vi "Solver LLB Pre-Check.vi"(8 "error in":errorcluster, 11 "Solver LLB":path) -> (0 "error out":errorcluster, 3 "Issues Detected":string)   [LabVIEW 2020]
uses:
  <vilib>/Utility/traverseref.llb/TRef TravTarget.ctl
  c793339f-25fd-4173-b65a-4e1b08b07bf6.vi
  1ab69464-b1f4-4e58-a4b1-b8e24fb308a9.vi
  <vilib>/Utility/traverseref.llb/VI Scripting - Traverse.lvlib
panel:
  in  "Prohibited Libraries":string[](array[string])=["Skyline", "registry"]
  in  "Prohibited Nodes":string[](array[string])=["Open VI Reference", "Call Library Function Node", "Traverse for GObjects.vi", "TCP Write", "TCP Read", "Call Chain", "Python Node", "Constructor Node", "Automation Open", "System Exec.vi", "Delete", "Librarian Delete.vi", "Delete Directory Recursive.vi", "Read Multiple Elements from Stream", "Read Single Element from Stream", "Write Multiple Elements to Stream", "Write Single Element to Stream", "VISA Write", "VISA Read", "DataSocket Read", "DataSocket Write"]
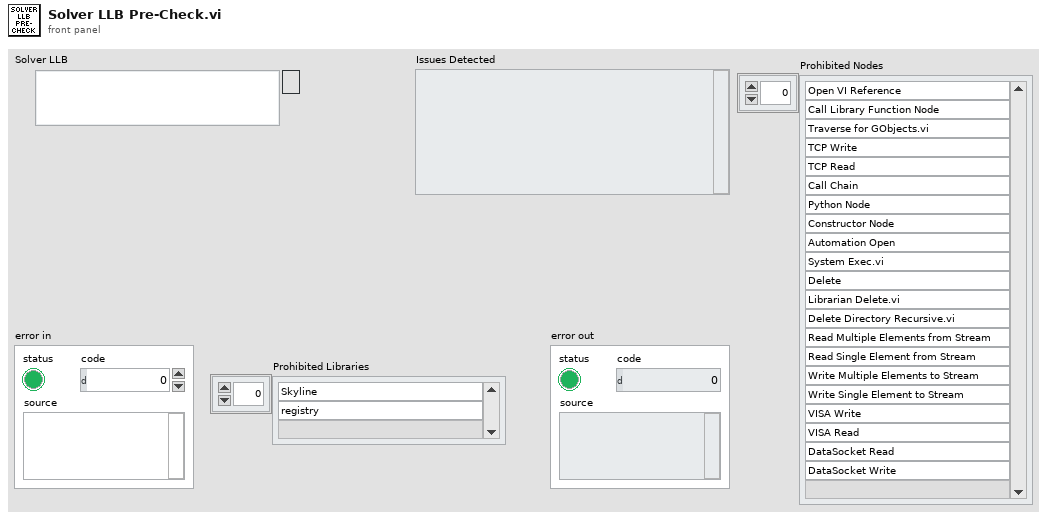
[diagram p1: front panel]
types:
  T1 = enum16{"Initialize", "Password-Protection", "Prohibited Nodes", "Prohibited Libraries", "Close"}
  T2 = enum16{"Initialize", "Password-Protection", "Prohibited Nodes", "Prohibited Libraries", "Close"}[]
  T3 = enum32{"invalid lock state", "Not Locked", "Locked (No Password)", "Password-protected"}
  T4 = typedef "TRef TravTarget.ctl" = enum16{"FP", "BD", "Other"}
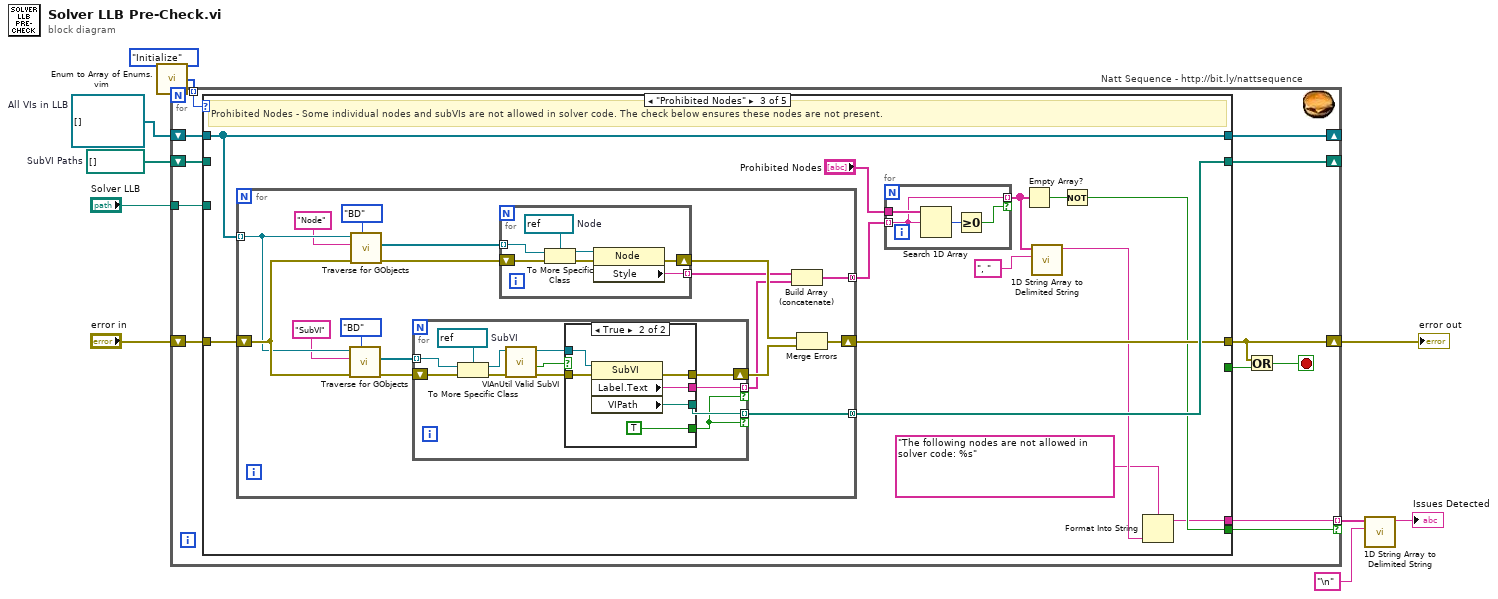
[diagram p0: block diagram]
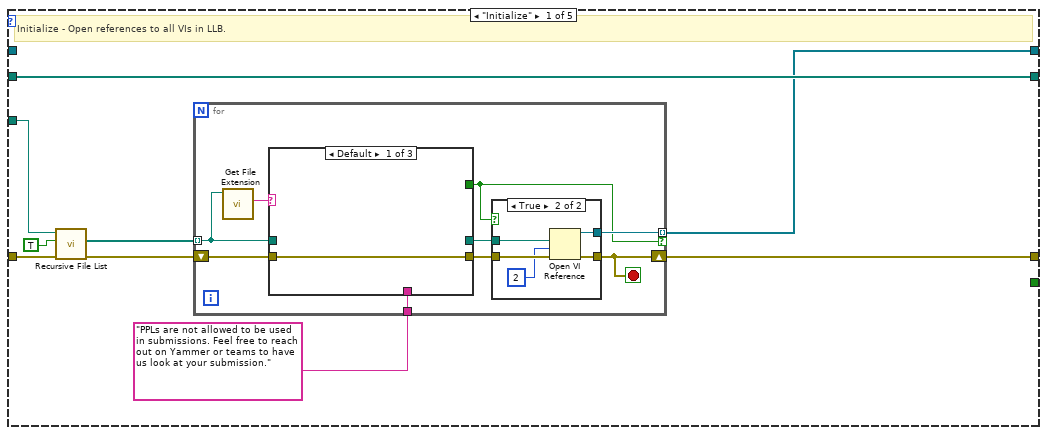
[diagram p2: hidden frame]
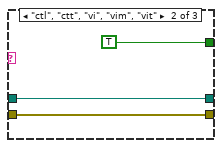
[diagram p4: hidden frame]
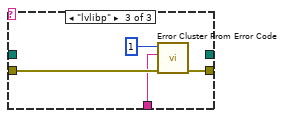
[diagram p5: hidden frame]
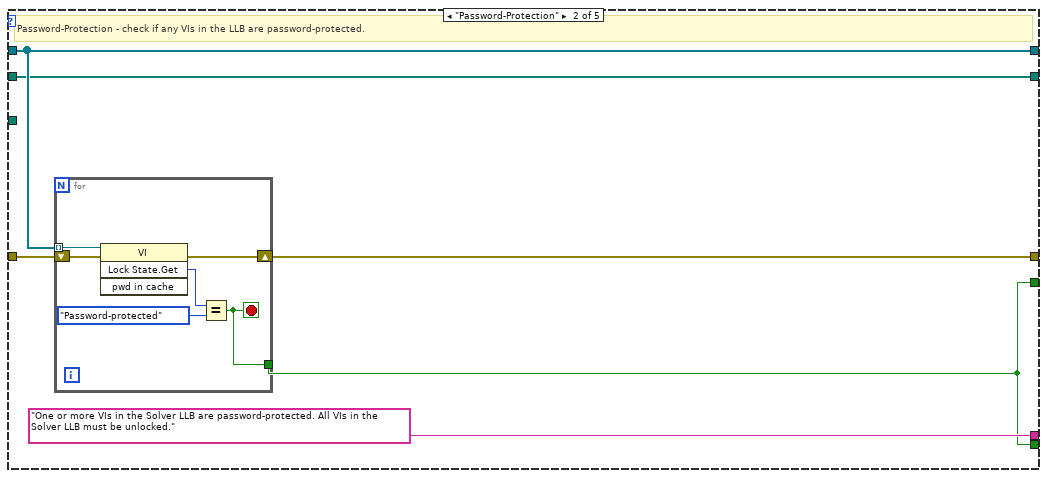
[diagram p6: hidden frame]
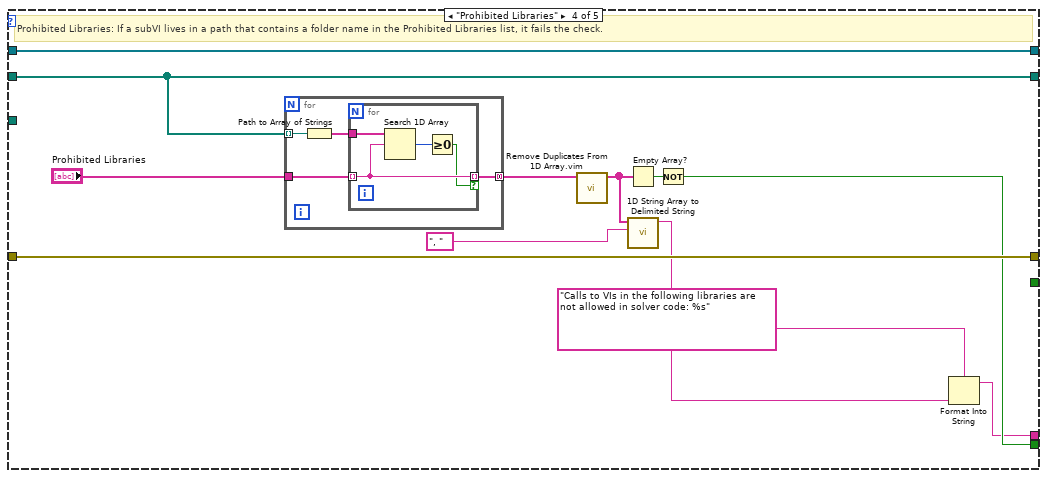
[diagram p8: hidden frame]
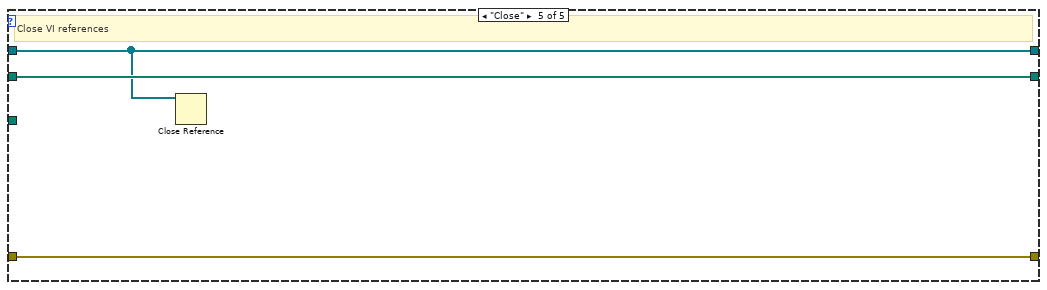
[diagram p9: hidden frame]
diagram:
  w1 = path[] []  # SubVI Paths
  w5 = refnum<vi>[] []  # All VIs in LLB
  n1 = call "Enum to Array of Enums.vim"("enum"=T1."Initialize") -> ("array of enums"=w10:T2)
  n2 = for "Natt Sequence - http://bit.ly/nattsequence" {
    tunnel: w10 -> [w22] mode=indexing
    tunnel: "Solver LLB" -> [w20]
    shift-right: [w13] -> w6
    shift-left: "error in" -> [w21]
    shift-right: [w19] -> _
    shift-left: w5 -> [w18]
    tunnel: [w17] -> w4 mode=indexing if=w16
    shift-right: [w15] -> _
    shift-left: w1 -> [w14]
    stop <- w12 stop-if-true
    n3 = case shown="\"Prohibited Nodes\"" w22 {
      tunnel: w21 -> [w31 w60 w79 w138 w149]
      tunnel: w20 -> [w30 _ _ _ _]
      tunnel: [w26 w58 w76 w138 w149] -> w13
      tunnel: [w24 w59 w78 w137 w147] -> w19
      tunnel: w18 -> [_ w59 w78 w137 w147]
      tunnel: [_ "One or more VIs in the Solver LLB are password-protected. All VIs in the Solver LLB must be unlocked." w69 w127 _] -> w17
      tunnel: [_ w55 w72 w130 _] -> w16
      tunnel: [w25 w56 w77 w136 w148] -> w15
      tunnel: w14 -> [w25 w56 _ w136 w148]
      tunnel: [_ w55 _ _ _] -> w11
      frame "Initialize" {
        # "Initialize - Open references to all VIs in LLB."
        n4 = call <vilib>:"Recursive File List.vi"("error in (no error)"=w31, "Treat LLBs as Folders?"=TRUE, "Folder Path"=w30) -> ("error out"=w28:errorcluster, "All Files in Dir"=w27:path[])  [unwired: 4 in, 3 out]
        n5 = for {
          shift-right: [w37] -> w26
          shift-left: w28 -> [w36]
          tunnel: w27 -> [w35] mode=indexing
          tunnel: [w40] -> w24 mode=indexing if=w38
          tunnel: "PPLs are not allowed to be used in submissions. Feel free to reach out on Yammer or teams to have us look at your submission." ("error message (\"\")") -> [w32]
          stop <- w37 stop-if-true
          n6 = call <vilib>:"Get File Extension.vi"("file"=w35) -> ("lowercase file extension"=w39:string)  [unwired: 6 in, 4 out]
          n7 = case shown="Default" w39 {
            tunnel: [_ TRUE _] -> w38
            tunnel: w36 -> [w47 w48 w54]
            tunnel: w35 -> [_ w49 _]
            tunnel: [_ w49 _] -> w34
            tunnel: [w47 w48 w53] -> w33
            tunnel: w32 -> [_ _ w51]
            frame Default {
            }
            frame "ctl", "ctt", "vi", "vim", "vit" {
            }
            frame "lvlibp" {
              n8 = call <vilib>:"Error Cluster From Error Code.vi"("error in (no error)"=w54, "error message (\"\")"=w51, "error code (0)"=1) -> ("error out"=w53:errorcluster)  [unwired: 6 in]
            }
          }
          n9 = case shown="True" w38 {
            tunnel: w33 -> [w41 w46]
            tunnel: [w41 w44] -> w37
            tunnel: [_ w43] -> w40
            tunnel: w34 -> [_ w42]
            frame False {
            }
            frame True {
              n10 = Open VI Reference(vi path=w42, options=2, error in (no error)=w46) -> (vi reference=w43:refnum<vi>, error out=w44:errorcluster)  [unwired: 3 in]
            }
          }
        }
      }
      frame "Password-Protection" {
        # "Password-Protection - check if any VIs in the LLB are password-protected."
        n11 = for {
          shift-right: [w64] -> w58
          shift-left: w60 -> [w66]
          tunnel: w59 -> [w65] mode=indexing
          tunnel: [w61] -> w55
          stop <- w61 stop-if-true
          n12 = invoke class="VI" method="Lock State.Get"(reference=w65, error in=w66) -> (error out=w64:errorcluster, "Get Lock State"=w63:T3)  [unwired: 2 in, 2 out]
          n13 = Equal?(x=w63, y=T3."Password-protected") -> (x = y?=w61:bool)
        }
      }
      frame "Prohibited Nodes" {
        # "Prohibited Nodes - Some individual nodes and subVIs are not allowed in solver code. The check below ensures these nodes are not present."
        n14 = for {
          shift-right: [w88] -> w76
          shift-left: w79 -> [w98]
          tunnel: w78 -> [w97] mode=indexing
          tunnel: [w87] -> w77 mode=concatenating
          tunnel: [w84] -> w74 mode=concatenating
          n15 = call <vilib>:"Traverse for GObjects.vi"("Traverse Target"=TRef_TravTarget."BD", "error in (no error)"=w98, "Class Name"="SubVI", "VI Refnum"=w97) -> ("error out"=w92:errorcluster, "References"=w91:refnum<vi>[])  [unwired: 4 in, 2 out]
          n16 = call <vilib>:"Traverse for GObjects.vi"("Traverse Target"=TRef_TravTarget."BD", "error in (no error)"=w98, "Class Name"="Node", "VI Refnum"=w97) -> ("error out"=w94:errorcluster, "References"=w93:refnum<vi>[])  [unwired: 4 in, 2 out]
          n17 = for {
            shift-right: [w109] -> w89
            shift-left: w92 -> [w112]
            tunnel: w91 -> [w111] mode=indexing
            tunnel: [w108] -> w85 mode=indexing if=w101
            tunnel: [w107] -> w87 mode=indexing if=w101
            w110 = refnum<vi> refnum  # SubVI
            n18 = To More Specific Class(target class=w110, reference=w111, error in=w112) -> (specific class reference=w104:refnum<vi>, error out=w106:errorcluster)
            n19 = call <vilib>:"VIAnUtil Valid SubVI.vi"("error in (no error)"=w106, "SubVI in"=w104) -> ("error out"=w105:errorcluster, "Valid SubVI?"=w102:bool, "SubVI out"=w103:refnum<vi>)  [unwired: 7 in]
            n20 = case shown="True" w102 {
              tunnel: [w113 w119] -> w109
              tunnel: [_ w118] -> w108
              tunnel: [_ w117] -> w107
              tunnel: w105 -> [w113 w116]
              tunnel: w103 -> [_ w115]
              tunnel: [_ TRUE] -> w101
              frame False {
              }
              frame True {
                n21 = property class="SubVI"(reference=w115, error in=w116) -> (error out=w119:errorcluster, "Label.Text"=w118:string, "VIPath"=w117:path)  [unwired: 1 out]
              }
            }
          }
          n22 = for {
            shift-right: [w121] -> w90
            shift-left: w94 -> [w126]
            tunnel: w93 -> [w125] mode=indexing
            tunnel: [w120] -> w86 mode=indexing
            w124 = refnum<vi> refnum  # Node
            n23 = To More Specific Class(target class=w124, reference=w125, error in=w126) -> (specific class reference=w123:refnum<vi>, error out=w122:errorcluster)
            n24 = property class="Node"(reference=w123, error in=w122) -> (error out=w121:errorcluster, "Style"=w120:string)  [unwired: 1 out]
          }
          n25 = Build Array (concatenate)(w86, w85) -> (w84:string[])
          n26 = Merge Errors(w90, w89) -> (w88:errorcluster)
        }
        n27 = for {
          tunnel: "Prohibited Nodes" -> [w83]
          tunnel: w74 -> [w82] mode=indexing
          tunnel: [w82] -> w71 mode=indexing if=w80
          n28 = Search 1D Array(1D array=w83, element=w82) -> (index of element=w81:i32)  [unwired: 1 in]
          n29 = Greater Or Equal To 0?(x=w81) -> (x >= 0?=w80:bool)
        }
        n30 = Empty Array?(array=w71) -> (empty?=w73:bool)
        n31 = call <vilib>:"1D String Array to Delimited String.vi"("delimiter"=", ", "string array"=w71) -> ("delimited string"=w68:string)  [unwired: 9 in]
        n32 = Not(x=w73) -> (.not. x?=w72:bool)
        n33 = Format Into String(format string="The following nodes are not allowed in solver code: %s", w68) -> (resulting string=w69:string)  [unwired: 2 in, 1 out]
      }
      frame "Prohibited Libraries" {
        # "Prohibited Libraries: If a subVI lives in a path that contains a folder name in the Prohibited Libraries list, it fails the check."
        n34 = for {
          tunnel: w136 -> [w142] mode=indexing
          tunnel: "Prohibited Libraries" -> [w141]
          tunnel: [w139] -> w134 mode=concatenating
          n35 = Path to Array of Strings(0:w142) -> (2:w140:string[])  [unwired: 1 out]
          n36 = for {
            tunnel: w141 -> [w144] mode=indexing
            tunnel: w140 -> [w146]
            tunnel: [w144] -> w139 mode=indexing if=w143
            n37 = Search 1D Array(1D array=w146, element=w144) -> (index of element=w145:i32)  [unwired: 1 in]
            n38 = Greater Or Equal To 0?(x=w145) -> (x >= 0?=w143:bool)
          }
        }
        n39 = call "Remove Duplicates From 1D Array.vim"("array"=w134) -> ("array with duplicates removed"=w131:string[])  [unwired: 10 in]
        n40 = Empty Array?(array=w131) -> (empty?=w133:bool)
        n41 = call <vilib>:"1D String Array to Delimited String.vi"("delimiter"=", ", "string array"=w131) -> ("delimited string"=w128:string)  [unwired: 9 in]
        n42 = Not(x=w133) -> (.not. x?=w130:bool)
        n43 = Format Into String(format string="Calls to VIs in the following libraries are not allowed in solver code: %s", w128) -> (resulting string=w127:string)  [unwired: 2 in, 1 out]
      }
      frame "Close" {
        # "Close VI references"
        n44 = Close Reference(reference=w147) -> ()  [unwired: 1 in, 1 out]
      }
    }
    n45 = Or(x=w13, y=w11) -> (x .or. y?=w12:bool)
  }
  "error out" <- w6
  n46 = call <vilib>:"1D String Array to Delimited String.vi"("delimiter"="\n", "string array"=w4) -> ("delimited string"=→"Issues Detected":string)  [unwired: 9 in]
